vi "2Dsave_bin_BD_MultiVessel_Ver12.vi"(8 "Error In":errorcluster, 9 "Number of B-scans":i32, 10 "refnum in":refnum<file>, 11 "queue in":refnum<queue>) -> (0 "error out":errorcluster, 2 "double precision float":dbl, 3 "prepend array or string size? (T)":bool)   [LabVIEW 2017]
panel:
  out "Acquired Buffer Number":dbl
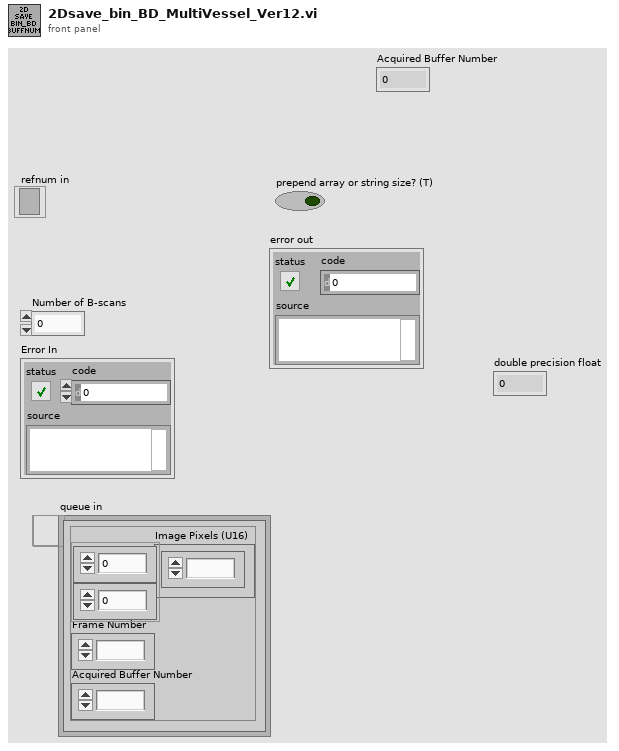
[diagram p1: front panel]
types:
  T1 = enum16{"big-endian, network order", "native, host order", "little-endian"}
  T2 = cluster{"Image Pixels (U16)":u16[][], "Frame Number":dbl, "Acquired Buffer Number":dbl}
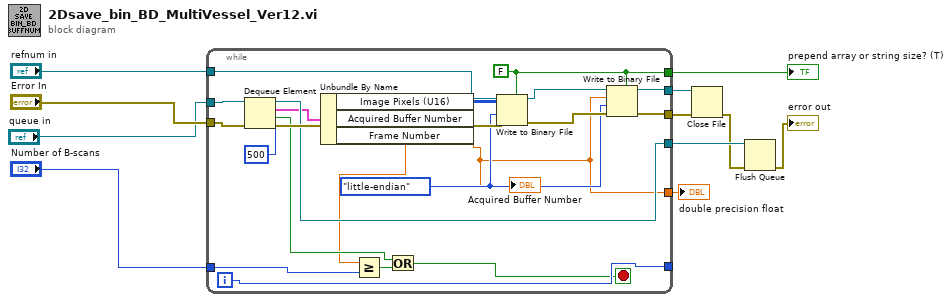
[diagram p0: block diagram]
diagram:
  n1 = while {
    tunnel: "queue in" -> [w14]
    tunnel: "Error In" -> [w13]
    tunnel: "refnum in" -> [w26]
    tunnel: [w23] -> w8
    tunnel: [w31] -> w11
    tunnel: "Number of B-scans" -> [w30]
    tunnel: [w20] -> w6
    tunnel: [w19] -> w5
    tunnel: [w15] -> w2
    tunnel: [w17] -> _
    i -> [w17]
    stop <- w16 stop-if-true
    w24 = T1."little-endian" ("byte order (0:big-endian, network order)")
    w23 = FALSE ("prepend array or string size? (T)")
    n2 = Dequeue Element(queue=w14, timeout in ms (-1)=500, error in (no error)=w13) -> (queue out=w31:refnum<queue>, element=w22:T2, timed out?=w28:bool, error out=w32:errorcluster)
    n3 = Unbundle By Name(w22) -> ("Image Pixels (U16)"=w21:u16[][], "Acquired Buffer Number"=w15:dbl, "Frame Number"=w12:dbl)
    "Acquired Buffer Number" <- w15
    n4 = Greater Or Equal?(x=w12, y=w30) -> (x >= y?=w29:bool)
    n5 = Or(x=w28, y=w29) -> (x .or. y?=w16:bool)
    n6 = Write to Binary File(file (use dialog)=w26, data=w21, error in=w32, 5:w23, 9:w24) -> (refnum out=w25:refnum<file>, error out=w27:errorcluster)  [unwired: 1 in, 1 out]
    n7 = Write to Binary File(file (use dialog)=w25, data=w15, error in=w27, 5:w23, 9:w24) -> (refnum out=w19:refnum<file>, error out=w20:errorcluster)  [unwired: 1 in, 1 out]
  }
  "prepend array or string size? (T)" <- w8
  "double precision float" <- w2
  n8 = Close File(refnum=w5, error in=w6) -> (error out=w9:errorcluster)  [unwired: 1 out]
  n9 = Flush Queue(queue=w11, error in (no error)=w9) -> (error out=→"error out":errorcluster)  [unwired: 2 out]
